vi "SinglePulse.vi"(8 "Stop heat (s)":dbl=10.0, 9 "Start heat (s)":dbl=5.0, 10 "Pulse Height (A) 2":dbl=1e-05) -> (0 "Power":dbl[](array[numeric]), 1 "Sample temperatur":dbl[](array[numeric]), 2 "Bath Temperature":dbl[](array[numeric]), 3 "Time":i32[](array[numeric]), 4 "XY Graph":cluster{dbl[], dbl[]}[](graph))   [LabVIEW 2019]
uses:
  Monitors/Utility/Monitor Communication/AMI/AMI_Control.ctl
  Global/Global Variables/Heat_global_variables.vi
  Instrument_Setup.vi
  Global/Global Variables/Data_Display_global.vi
  Monitors/Utility/Monitor Communication/sub-vis/K6221_Open_Queue.vi
  Global/Global Variables/global.vi
  Equipment/Lake Shore 372/Lake Shore 372.lvlib
  Equipment/Keithley 2182/Keithley 2182.lvlib
panel:
  out "Current":dbl[](array[numeric])
  out "Voltage":dbl[](array[numeric])
  out "Indices":u32[](array[numeric])
  out "W":dbl
  out "R2":dbl
  out "R1":dbl
  out "T2":dbl
  out "T1":dbl
  out "A":dbl
  out "V":dbl
  out "Was K2182A-Monitor activatet?":bool
  out "Was LS372_readout-Monitor activatet?":bool
  out "Was LS370_readout-Monitor activatet?":bool
  out "Relax":bool
  out "Heat":bool
  out "Stabilize":bool
  # "current values"
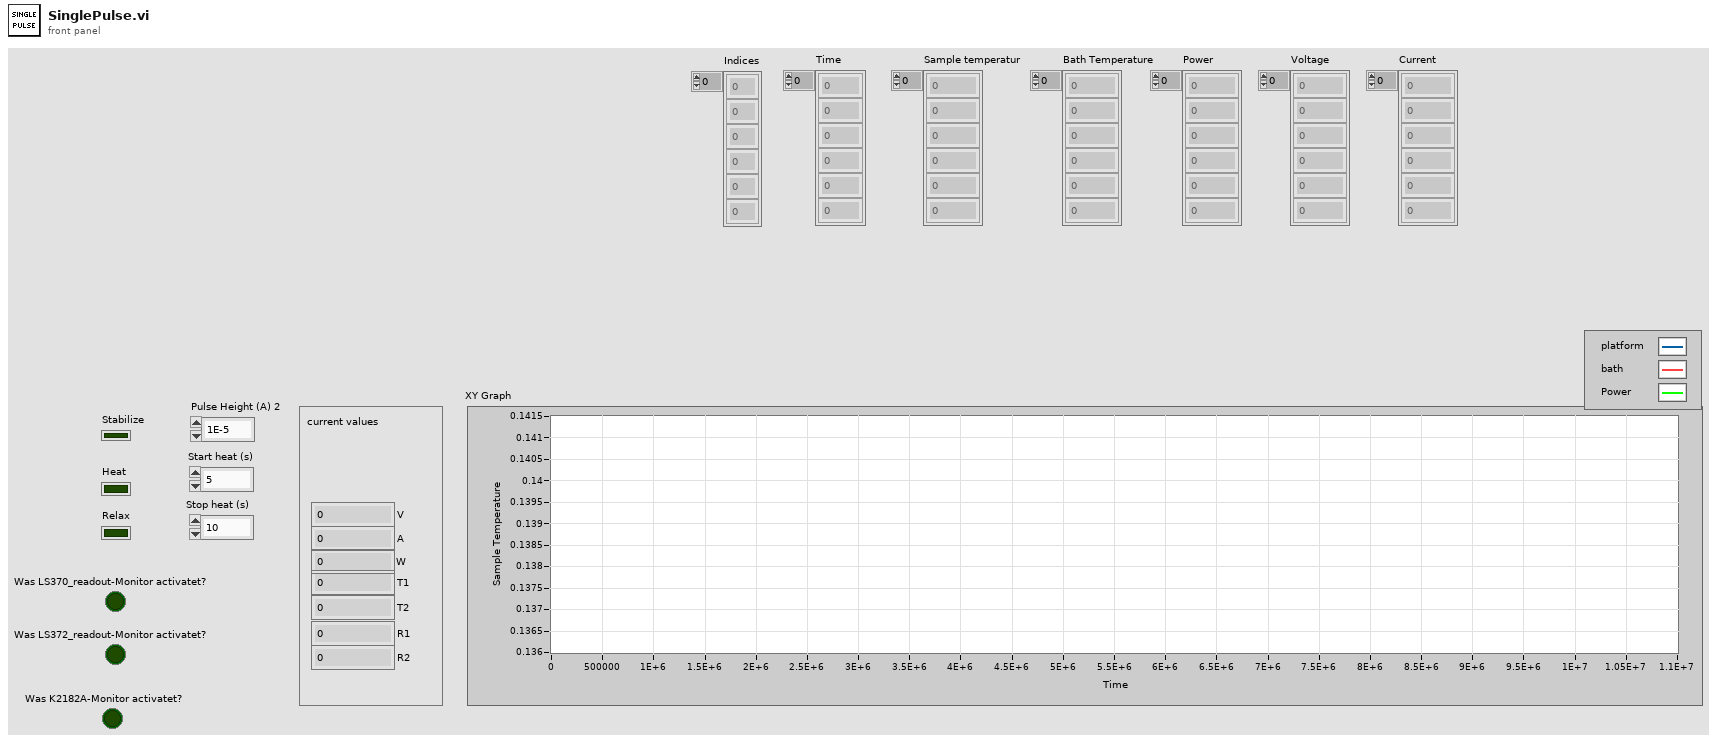
[diagram p1: front panel]
types:
  T1 = cluster{"Lakeshore 370 ":refnum<visa-resource-name>, "Lakeshore 372":refnum<visa-resource-name>, "Platform Channel":i32, "Bath Channel ":i32, "Platform Temperature Control":u16, "Bath Temperature Control":u16}
  T2 = cluster{"VISA Keithley 2182A":refnum<visa-resource-name>, "Measurement (0: Voltage Channel 1)":i32, "Integration Rate (5)":dbl, "Integration Rate Units (0: Line Cycles)":i32, "Sample Count (1)":i32, "Voltage Resolution (8)":i32, "Enable Ratio (F: Disable)":bool, "Enable Delta (F: Disable)":bool, "Enable Analog Filter (T: Enable)":bool, "Enable Digital Filter (T: Enable)":bool, "Filter Window (0.01%)":dbl, "Filter Count (10)":i32, "Filter Type (0: Moving)":i32}
  T3 = typedef "AMI_Control.ctl" = cluster{"B Rate (T/min)":dbl, "B Setpoint (T)":dbl, "Phi Setpoint (Deg)":dbl, "Set Persistent":bool, "Update":bool}
  T4 = typedef "K6221_Cluster.ctl" = cluster{"Plot Window":dbl[][], "A":dbl, "A (RMS)":dbl, "Hz":dbl, "I (A)":dbl, "f (Hz)":dbl, "Update":bool, "Offset":dbl, "Offset (A)":dbl, "Compliance":bool, "Output":bool, "Output Status":bool}
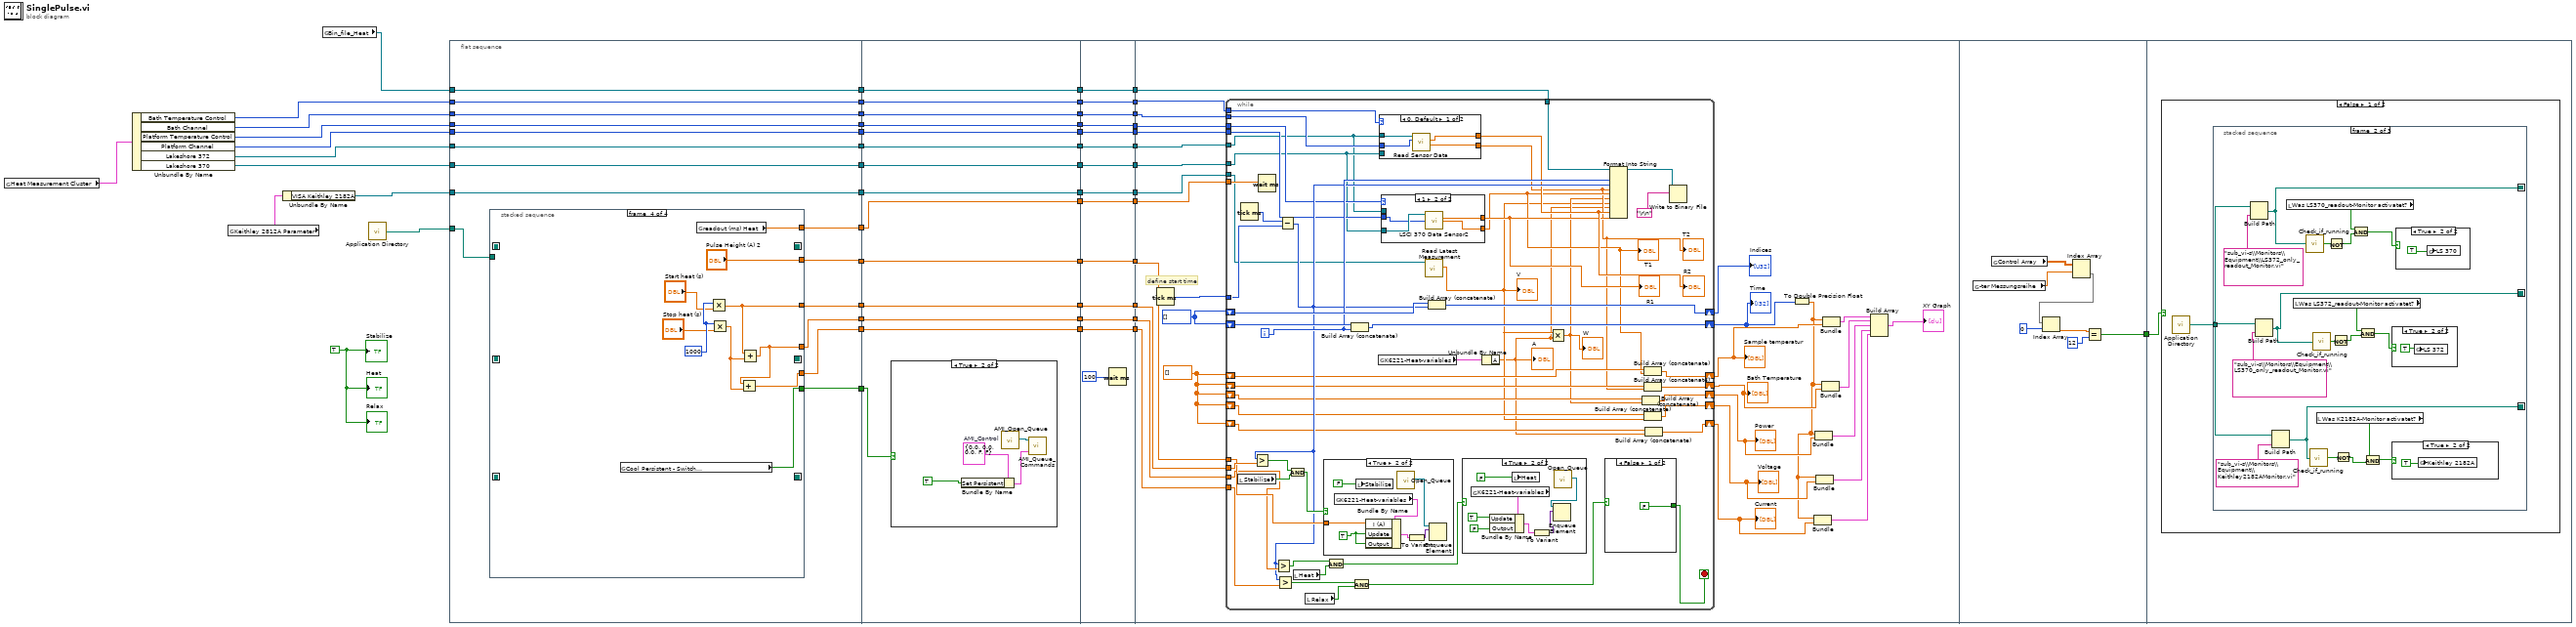
[diagram p0: block diagram]
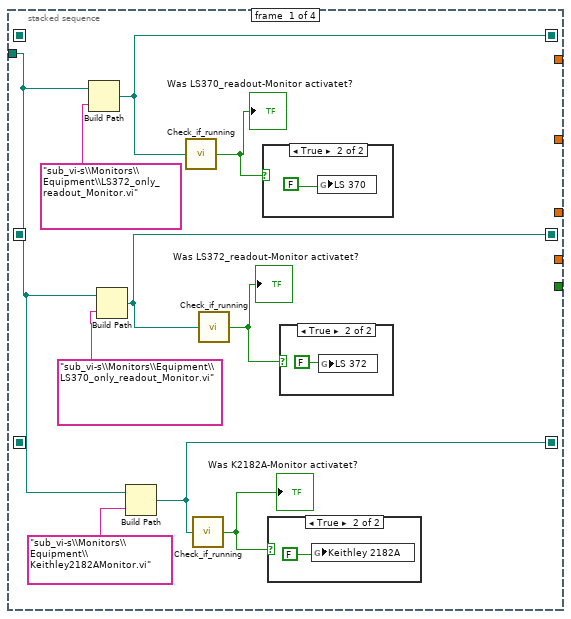
[diagram p2: hidden frame]
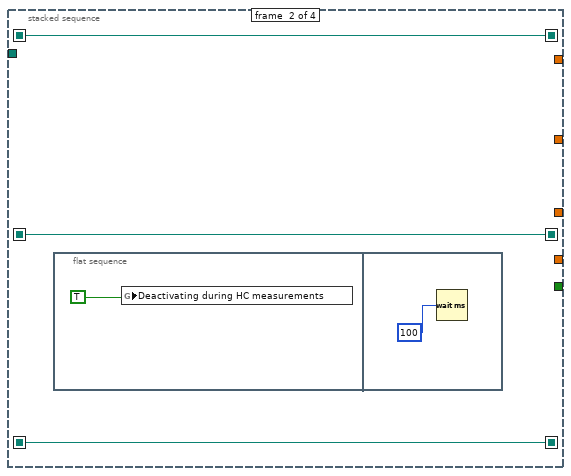
[diagram p6: hidden frame]
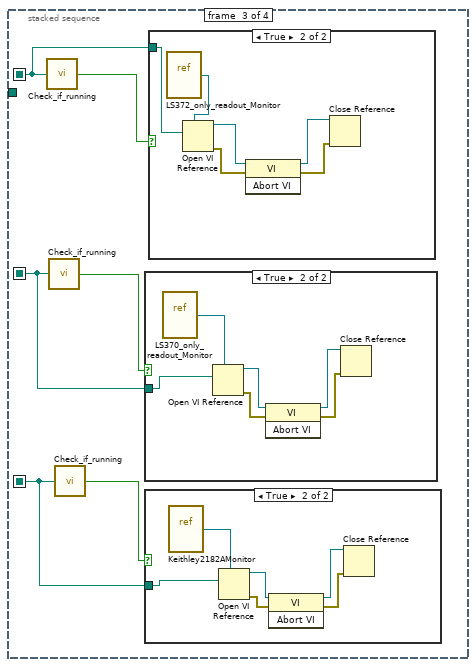
[diagram p7: hidden frame]
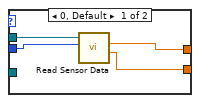
[diagram p12: hidden frame]
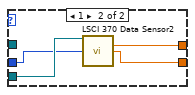
[diagram p13: hidden frame]
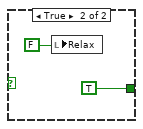
[diagram p14: hidden frame]
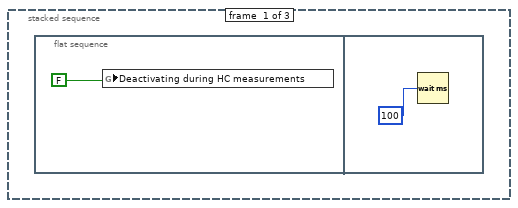
[diagram p17: hidden frame]
diagram:
  w50 = TRUE
  n1 = global read "Instrument_Setup.vi" "Heat Measurement Cluster"() -> (w19:T1)
  n2 = Unbundle By Name(w19) -> ("Bath Temperature Control"=w12:u16, "Bath Channel"=w13:i32, "Platform Temperature Control"=w15:u16, "Platform Channel"=w16:i32, "Lakeshore 372"=w17:refnum<visa-resource-name>, "Lakeshore 370"=w18:refnum<visa-resource-name>)
  n3 = global read "Instrument_Setup.vi" "Keithley 2812A Parameter"() -> (w52:T2)
  n4 = Unbundle By Name(w52) -> ("VISA Keithley 2182A"=w51:refnum<visa-resource-name>)
  n5 = global read "Heat_global_variables.vi" "Bin_file_Heat"() -> (w53:refnum<file>)
  n6 = call <vilib>:"Application Directory.vi"() -> ("Application Directory"=w49:path)
  n7 = flat-sequence {
    tunnel: w53 -> [w67]
    tunnel: w17 -> [w66]
    tunnel: w18 -> [w65]
    tunnel: w51 -> [w64]
    tunnel: w49 -> [w68]
    tunnel: [w67] -> w48
    tunnel: [w66] -> w47
    tunnel: [w65] -> w46
    tunnel: [w64] -> w45
    tunnel: [w63] -> w44
    tunnel: [w62] -> w43
    tunnel: [w61] -> w42
    tunnel: [w60] -> w29
    tunnel: [w59] -> w26
    tunnel: [w58] -> w23
    tunnel: [w57] -> w20
    tunnel: w16 -> [w57]
    tunnel: w15 -> [w56]
    tunnel: [w56] -> w14
    tunnel: w13 -> [w54]
    tunnel: w12 -> [w55]
    tunnel: [w55] -> w11
    tunnel: [w54] -> w10
    tunnel: w48 -> [w133]
    tunnel: w47 -> [w132]
    tunnel: w46 -> [w131]
    tunnel: w45 -> [w130]
    tunnel: w44 -> [w129]
    tunnel: w43 -> [w128]
    tunnel: w42 -> [w134]
    tunnel: [w133] -> w41
    tunnel: [w132] -> w39
    tunnel: [w131] -> w37
    tunnel: [w130] -> w35
    tunnel: [w129] -> w33
    tunnel: [w128] -> w31
    tunnel: w29 -> [w127]
    tunnel: [w127] -> w27
    tunnel: w26 -> [w126]
    tunnel: [w126] -> w24
    tunnel: w23 -> [w125]
    tunnel: [w125] -> w21
    tunnel: w20 -> [w121]
    tunnel: w14 -> [w122]
    tunnel: w11 -> [w124]
    tunnel: w10 -> [w123]
    tunnel: [w124] -> w9
    tunnel: [w123] -> w8
    tunnel: [w122] -> w7
    tunnel: [w121] -> w6
    tunnel: w41 -> [w152]
    tunnel: [w152] -> w40
    tunnel: w39 -> [w151]
    tunnel: [w151] -> w38
    tunnel: w37 -> [w150]
    tunnel: [w150] -> w36
    tunnel: w35 -> [w149]
    tunnel: [w149] -> w34
    tunnel: w33 -> [w148]
    tunnel: [w148] -> w32
    tunnel: w31 -> [w147]
    tunnel: [w147] -> w30
    tunnel: [w145] -> w28
    tunnel: w27 -> [w145]
    tunnel: [w144] -> w25
    tunnel: w24 -> [w144]
    tunnel: [w143] -> w22
    tunnel: w21 -> [w143]
    tunnel: w9 -> [w142]
    tunnel: w8 -> [w141]
    tunnel: w7 -> [w140]
    tunnel: w6 -> [w139]
    tunnel: [w142] -> w5
    tunnel: [w141] -> w4
    tunnel: [w140] -> w3
    tunnel: [w139] -> w2
    tunnel: w40 -> [w182]
    tunnel: w38 -> [w181]
    tunnel: w36 -> [w180]
    tunnel: w34 -> [w179]
    tunnel: w32 -> [w175]
    tunnel: w30 -> [w174]
    tunnel: w28 -> [w173]
    tunnel: w25 -> [w172]
    tunnel: w22 -> [w171]
    tunnel: w5 -> [w170]
    tunnel: w4 -> [w169]
    tunnel: w3 -> [w168]
    tunnel: w2 -> [w167]
    tunnel: [w267] -> w1
    tunnel: w1 -> [w274]
    frame #0 {
      n8 = stacked-sequence {
        seq-local: [w71 _ _ _] -> [_ w84 _ _]
        seq-local: [w70 _ _ _] -> [_ w83 _ _]
        seq-local: [w69 _ _ _] -> [_ w82 _ _]
        seq-local: [_ w84 _ _] -> [_ _ w89 _]
        seq-local: [_ w83 _ _] -> [_ _ w88 _]
        seq-local: [_ w82 _ _] -> [_ _ w87 _]
        tunnel: w68 -> [w76 _ _ _]
        tunnel: [_ _ _ "Pulse Height (A) 2"] -> w63
        tunnel: [_ _ _ w112] -> w62
        tunnel: [_ _ _ w116] -> w61
        tunnel: [_ _ _ w114] -> w60
        tunnel: [_ _ _ w113] -> w59
        tunnel: [_ _ _ w111] -> w58
        frame #0 {
          n9 = Build Path(base path=w76, name or relative path="sub_vi-s\\Monitors\\Equipment\\LS372_only_readout_Monitor.vi") -> (appended path=w71:path)
          n10 = Build Path(base path=w76, name or relative path="sub_vi-s\\Monitors\\Equipment\\LS370_only_readout_Monitor.vi") -> (appended path=w70:path)
          n11 = Build Path(base path=w76, name or relative path="sub_vi-s\\Monitors\\Equipment\\Keithley2182AMonitor.vi") -> (appended path=w69:path)
          n12 = call "Check_if_running.vi"("VI-Pfad"=w71) -> ("Running"=w74:bool)
          "Was LS370_readout-Monitor activatet?" <- w74
          n13 = call "Check_if_running.vi"("VI-Pfad"=w69) -> ("Running"=w72:bool)
          "Was K2182A-Monitor activatet?" <- w72
          n14 = call "Check_if_running.vi"("VI-Pfad"=w70) -> ("Running"=w73:bool)
          "Was LS372_readout-Monitor activatet?" <- w73
          n15 = case shown="True" w74 {
            frame False {
            }
            frame True {
              n16 = global write "Instrument_Setup.vi" "LS 370"(FALSE) -> ()
            }
          }
          n17 = case shown="True" w72 {
            frame False {
            }
            frame True {
              n18 = global write "Instrument_Setup.vi" "Keithley 2182A"(FALSE) -> ()
            }
          }
          n19 = case shown="True" w73 {
            frame False {
            }
            frame True {
              n20 = global write "Instrument_Setup.vi" "LS 372"(FALSE) -> ()
            }
          }
        }
        frame #1 {
          n21 = flat-sequence {
            frame #0 {
              n22 = global write "Data_Display_global.vi" "Deactivating during HC measurements"(TRUE) -> ()
            }
            frame #1 {
              n23 = Wait (ms)(milliseconds to wait=100) -> ()  [unwired: 1 out]
            }
          }
        }
        frame #2 {
          n24 = call "Check_if_running.vi"("VI-Pfad"=w89) -> ("Running"=w92:bool)
          n25 = call "Check_if_running.vi"("VI-Pfad"=w88) -> ("Running"=w91:bool)
          n26 = call "Check_if_running.vi"("VI-Pfad"=w87) -> ("Running"=w90:bool)
          n27 = case shown="True" w91 {
            tunnel: w88 -> [_ w104]
            frame False {
            }
            frame True {
              n28 = vi-ref "LS370_only_readout_Monitor.vi"() -> (w103:refnum<vi>)
              n29 = Open VI Reference(type specifier VI Refnum (for type only)=w103, vi path=w104) -> (vi reference=w102:refnum<vi>, error out=w101:errorcluster)  [unwired: 4 in]
              n30 = invoke class="VI" method="Abort VI"(reference=w102, error in=w101) -> (reference out=w100:refnum<vi>, error out=w99:errorcluster)  [unwired: 1 in, 1 out]
              n31 = Close Reference(reference=w100, error in (no error)=w99) -> ()  [unwired: 1 out]
            }
          }
          n32 = case shown="True" w90 {
            tunnel: w87 -> [_ w98]
            frame False {
            }
            frame True {
              n33 = vi-ref "Keithley2182AMonitor.vi"() -> (w97:refnum<vi>)
              n34 = Open VI Reference(type specifier VI Refnum (for type only)=w97, vi path=w98) -> (vi reference=w96:refnum<vi>, error out=w95:errorcluster)  [unwired: 4 in]
              n35 = invoke class="VI" method="Abort VI"(reference=w96, error in=w95) -> (reference out=w94:refnum<vi>, error out=w93:errorcluster)  [unwired: 1 in, 1 out]
              n36 = Close Reference(reference=w94, error in (no error)=w93) -> ()  [unwired: 1 out]
            }
          }
          n37 = case shown="True" w92 {
            tunnel: w89 -> [_ w109]
            frame False {
            }
            frame True {
              n38 = vi-ref "LS372_only_readout_Monitor.vi"() -> (w110:refnum<vi>)
              n39 = Open VI Reference(type specifier VI Refnum (for type only)=w110, vi path=w109) -> (vi reference=w108:refnum<vi>, error out=w107:errorcluster)  [unwired: 4 in]
              n40 = invoke class="VI" method="Abort VI"(reference=w108, error in=w107) -> (reference out=w106:refnum<vi>, error out=w105:errorcluster)  [unwired: 1 in, 1 out]
              n41 = Close Reference(reference=w106, error in (no error)=w105) -> ()  [unwired: 1 out]
            }
          }
        }
        frame #3 {
          w120 = 1000
          n42 = global read "Instrument_Setup.vi" "Cool Persistent - Switch\n during measurement"() -> (w116:bool)
          n43 = global read "Instrument_Setup.vi" "readout (ms) Heat"() -> (w111:dbl)
          n44 = Multiply(x=w120, y="Start heat (s)") -> (x*y=w112:dbl)
          n45 = Multiply(x=w120, y="Stop heat (s)") -> (x*y=w115:dbl)
          n46 = Add(x=w112, y=w115) -> (x+y=w114:dbl)
          n47 = Add(x=w114, y=w115) -> (x+y=w113:dbl)
        }
      }
    }
    frame #1 {
      n48 = case shown="True" w134 {
        frame False {
        }
        frame True {
          w136 = T3 {"B Rate (T/min)"=0.0, "B Setpoint (T)"=0.0, "Phi Setpoint (Deg)"=0.0, "Set Persistent"=FALSE, "Update"=FALSE}  # AMI_Control
          n49 = Bundle By Name(cluster=w136, "Set Persistent"=TRUE) -> (w137:T3)
          n50 = call "AMI_Open_Queue.vi"() -> ("queue out"=w138:refnum<queue>)  [unwired: 10 in, 1 out]
          n51 = call "AMI_Queue_Commands.vi"("AMI_Control"=w137, "Queue in"=w138) -> ()  [unwired: 1 in, 1 out]
        }
      }
    }
    frame #2 {
      n52 = Wait (ms)(milliseconds to wait=100) -> ()  [unwired: 1 out]
    }
    frame #3 {
      w177 = i32[] []
      w176 = dbl[] []
      # "define start time"
      n53 = Tick Count (ms)() -> (millisecond timer value=w178:u32)
      n54 = while {
        tunnel: w182 -> [w214]
        tunnel: w181 -> [w202]
        tunnel: w180 -> [w203]
        tunnel: w179 -> [w201]
        tunnel: w178 -> [w233]
        shift-right: [w231] -> w166
        shift-left: w177 -> [w232]
        shift-right: [w229] -> w165
        shift-left: w177 -> [w230]
        shift-right: [w196] -> w163
        shift-left: w176 -> [w197]
        shift-right: [w192] -> w162
        shift-left: w176 -> [w194]
        shift-right: [w190] -> w159
        shift-left: w176 -> [w191]
        shift-right: [w188] -> w158
        shift-left: w176 -> [w187]
        shift-right: [w185] -> w156
        shift-left: w176 -> [w184]
        tunnel: w175 -> [w224]
        tunnel: w174 -> [w228]
        tunnel: w173 -> [w223]
        tunnel: w172 -> [w222]
        tunnel: w171 -> [w210]
        tunnel: w170 -> [w207]
        tunnel: w169 -> [w206]
        tunnel: w168 -> [w205]
        tunnel: w167 -> [w204]
        i -> [w209]
        stop <- w215 stop-if-true
        n55 = local read "Stabilize"() -> (w227:bool)
        n56 = Tick Count (ms)() -> (millisecond timer value=w211:u32)
        n57 = Wait (ms)(milliseconds to wait=w210) -> ()  [unwired: 1 out]
        n58 = Subtract(x=w211, y=w233) -> (x-y=w208:u32)
        n59 = Greater?(x=w208, y=w228) -> (0:w226:bool)
        n60 = Greater?(x=w208, y=w223) -> (0:w221:bool)
        n61 = Greater?(x=w208, y=w222) -> (0:w218:bool)
        n62 = And(x=w226, y=w227) -> (x .and. y?=w225:bool)
        n63 = local read "Heat"() -> (w220:bool)
        n64 = local read "Relax"() -> (w217:bool)
        n65 = case shown="True" w225 {
          tunnel: w224 -> [_ w264]
          frame False {
          }
          frame True {
            w263 = TRUE
            n66 = global read "Heat_global_variables.vi" "K6221-Heat-variables"() -> (w265:T4)
            n67 = local write "Stabilize"(FALSE) -> ()
            n68 = Bundle By Name(cluster=w265, "I (A)"=w264, "Update"=w263, "Output"=w263) -> (w262:T4)
            n69 = call-poly "Open_Queue.vi"() -> ("queue out"=w260:refnum<queue>)  [unwired: 10 in, 1 out]
            n70 = To Variant(anything=w262) -> (Variant=w261:variant)
            n71 = Enqueue Element(queue=w260, element=w261) -> ()  [unwired: 2 in, 3 out]
          }
        }
        n72 = And(x=w221, y=w220) -> (x .and. y?=w219:bool)
        n73 = Build Array (concatenate)(w230, w209) -> (w229:i32[])
        n74 = And(x=w218, y=w217) -> (x .and. y?=w216:bool)
        n75 = global read "Heat_global_variables.vi" "K6221-Heat-variables"() -> (w200:T4)
        n76 = case shown="0, Default" w207 {
          tunnel: w202 -> [w245 _]
          tunnel: w206 -> [w244 w248]
          tunnel: w203 -> [_ w249]
          tunnel: [w243 w247] -> w199
          tunnel: [w242 w246] -> w193
          frame 0, Default {
            n77 = call "Read Sensor Data.vi"("Channel (1:1)"=w244, "VISA resource name"=w245) -> ("Kelvin Reading"=w242:dbl, "Resistance Reading"=w243:dbl)  [unwired: 4 in, 4 out]
          }
          frame 1 {
            n78 = call "LSCI 370 Data Sensor2.vi"("VISA session"=w249, "Channel (1)"=w248) -> ("Resistance Reading"=w247:dbl, "Kelvin Reading"=w246:dbl)  [unwired: 9 in, 3 out]
          }
        }
        "T2" <- w193
        "R2" <- w199
        n79 = case shown="1" w205 {
          tunnel: w204 -> [w236 w240]
          tunnel: w203 -> [_ w241]
          tunnel: [w235 w239] -> w198
          tunnel: [w234 w238] -> w195
          tunnel: w202 -> [w237 _]
          frame 0, Default {
            n80 = call "Read Sensor Data.vi"("Channel (1:1)"=w236, "VISA resource name"=w237) -> ("Kelvin Reading"=w234:dbl, "Resistance Reading"=w235:dbl)  [unwired: 4 in, 4 out]
          }
          frame 1 {
            n81 = call "LSCI 370 Data Sensor2.vi"("VISA session"=w241, "Channel (1)"=w240) -> ("Resistance Reading"=w239:dbl, "Kelvin Reading"=w238:dbl)  [unwired: 9 in, 3 out]
          }
        }
        "T1" <- w195
        "R1" <- w198
        n82 = call "Read Latest Measurement.vi"("VISA resource name"=w201) -> ("Measurement"=w186:dbl)  [unwired: 7 in, 3 out]
        "V" <- w186
        n83 = Build Array (concatenate)(w232, w208) -> (w231:u32[])
        n84 = case shown="True" w219 {
          frame False {
          }
          frame True {
            n85 = global read "Heat_global_variables.vi" "K6221-Heat-variables"() -> (w258:T4)
            n86 = Bundle By Name(cluster=w258, "Update"=TRUE, "Output"=FALSE) -> (w254:T4)
            n87 = local write "Heat"(FALSE) -> ()
            n88 = To Variant(anything=w254) -> (Variant=w253:variant)
            n89 = call-poly "Open_Queue.vi"() -> ("queue out"=w255:refnum<queue>)  [unwired: 10 in, 1 out]
            n90 = Enqueue Element(queue=w255, element=w253) -> ()  [unwired: 2 in, 3 out]
          }
        }
        n91 = Unbundle By Name(w200) -> ("A"=w183:dbl)
        "A" <- w183
        n92 = Multiply(x=w186, y=w183) -> (x*y=w189:dbl)
        "W" <- w189
        n93 = case shown="False" w216 {
          tunnel: [FALSE TRUE] -> w215
          frame False {
          }
          frame True {
            n94 = local write "Relax"(FALSE) -> ()
          }
        }
        n95 = Format Into String(initial string=w214, w209, w208, w193, w195, w189, w186, w183, w199, w198) -> (resulting string=w213:refnum<file>)  [unwired: 2 in, 1 out]
        n96 = Build Array (concatenate)(w191, w189) -> (w190:dbl[])
        n97 = Build Array (concatenate)(w194, w193) -> (w192:dbl[])
        n98 = Build Array (concatenate)(w187, w186) -> (w188:dbl[])
        n99 = Build Array (concatenate)(w197, w195) -> (w196:dbl[])
        n100 = Build Array (concatenate)(w184, w183) -> (w185:dbl[])
        n101 = Write to Binary File(file (use dialog)=w213, data="\r\n") -> ()  [unwired: 4 in, 3 out]
      }
      "Indices" <- w166
      "Sample temperatur" <- w163
      "Time" <- w165
      "Bath Temperature" <- w162
      "Power" <- w159
      "Voltage" <- w158
      "Current" <- w156
      n102 = To Double Precision Float(number=w165) -> (double precision float=w155:dbl[])
      n103 = Bundle(w155, w156) -> (w154:cluster{dbl[], dbl[]})  [unwired: 1 in]
      n104 = Bundle(w155, w159) -> (w160:cluster{dbl[], dbl[]})  [unwired: 1 in]
      n105 = Bundle(w155, w158) -> (w157:cluster{dbl[], dbl[]})  [unwired: 1 in]
      n106 = Bundle(w155, w162) -> (w161:cluster{dbl[], dbl[]})  [unwired: 1 in]
      n107 = Bundle(w155, w163) -> (w164:cluster{dbl[], dbl[]})  [unwired: 1 in]
      n108 = Build Array(w164, w161, w160, w157, w154) -> (→"XY Graph":cluster{dbl[], dbl[]}[])
    }
    frame #4 {
      n109 = global read "global.vi" "-ter Messungsreihe"() -> (w273:dbl)
      n110 = global read "global.vi" "Control Array"() -> (w271:dbl[][])
      n111 = Index Array(array=w271, index (row)=w273) -> (element=w272:dbl[])  [unwired: 1 in]
      n112 = Index Array(array=w272, index=0) -> (element=w269:dbl)
      n113 = Equal?(x=w269, y=12) -> (x = y?=w267:bool)
    }
    frame #5 {
      n114 = case shown="False" w274 {
        frame False {
          n115 = call <vilib>:"Application Directory.vi"() -> ("Application Directory"=w275:path)
          n116 = stacked-sequence {
            seq-local: [_ w292 _] -> [_ _ w305]
            seq-local: [_ w291 _] -> [_ _ w303]
            seq-local: [_ w290 _] -> [_ _ w301]
            tunnel: w275 -> [_ w293 _]
            frame #0 {
              n117 = flat-sequence {
                frame #0 {
                  n118 = global write "Data_Display_global.vi" "Deactivating during HC measurements"(FALSE) -> ()
                }
                frame #1 {
                  n119 = Wait (ms)(milliseconds to wait=100) -> ()  [unwired: 1 out]
                }
              }
            }
            frame #1 {
              n120 = Build Path(base path=w293, name or relative path="sub_vi-s\\Monitors\\Equipment\\LS372_only_readout_Monitor.vi") -> (appended path=w292:path)
              n121 = Build Path(base path=w293, name or relative path="sub_vi-s\\Monitors\\Equipment\\LS370_only_readout_Monitor.vi") -> (appended path=w291:path)
              n122 = Build Path(base path=w293, name or relative path="sub_vi-s\\Monitors\\Equipment\\Keithley2182AMonitor.vi") -> (appended path=w290:path)
              n123 = local read "Was LS370_readout-Monitor activatet?"() -> (w279:bool)
              n124 = local read "Was LS372_readout-Monitor activatet?"() -> (w283:bool)
              n125 = call "Check_if_running.vi"("VI-Pfad"=w292) -> ("Running"=w281:bool)
              n126 = call "Check_if_running.vi"("VI-Pfad"=w290) -> ("Running"=w288:bool)
              n127 = call "Check_if_running.vi"("VI-Pfad"=w291) -> ("Running"=w285:bool)
              n128 = local read "Was K2182A-Monitor activatet?"() -> (w286:bool)
              n129 = Not(x=w281) -> (.not. x?=w280:bool)
              n130 = Not(x=w285) -> (.not. x?=w284:bool)
              n131 = Not(x=w288) -> (.not. x?=w287:bool)
              n132 = And(x=w279, y=w280) -> (x .and. y?=w278:bool)
              n133 = And(x=w283, y=w284) -> (x .and. y?=w282:bool)
              n134 = And(x=w286, y=w287) -> (x .and. y?=w289:bool)
              n135 = case shown="True" w282 {
                frame False {
                }
                frame True {
                  n136 = global write "Instrument_Setup.vi" "LS 372"(TRUE) -> ()
                }
              }
              n137 = case shown="True" w289 {
                frame False {
                }
                frame True {
                  n138 = global write "Instrument_Setup.vi" "Keithley 2182A"(TRUE) -> ()
                }
              }
              n139 = case shown="True" w278 {
                frame False {
                }
                frame True {
                  n140 = global write "Instrument_Setup.vi" "LS 370"(TRUE) -> ()
                }
              }
            }
            frame #2 {
              n141 = global read "Instrument_Setup.vi" "LS 370"() -> (w304:bool)
              n142 = global read "Instrument_Setup.vi" "LS 372"() -> (w302:bool)
              n143 = global read "Instrument_Setup.vi" "Keithley 2182A"() -> (w300:bool)
              n144 = case shown="True" w304 {
                tunnel: w305 -> [_ w308]
                frame False {
                }
                frame True {
                  n145 = call "Start_Vi.vi"("VI-Pfad"=w308) -> ()  [unwired: 1 in]
                }
              }
              n146 = case shown="True" w302 {
                tunnel: w303 -> [_ w307]
                frame False {
                }
                frame True {
                  n147 = call "Start_Vi.vi"("VI-Pfad"=w307) -> ()  [unwired: 1 in]
                }
              }
              n148 = case shown="True" w300 {
                tunnel: w301 -> [_ w306]
                frame False {
                }
                frame True {
                  n149 = call "Start_Vi.vi"("VI-Pfad"=w306) -> ()  [unwired: 1 in]
                }
              }
            }
          }
        }
        frame True {
        }
      }
    }
  }
  "Stabilize" <- w50
  "Heat" <- w50
  "Relax" <- w50
